vi "Allow UI_Write.vi"(8 "error in (no error)":errorcluster, 10 "Allow UI?":bool=TRUE, 11 "Dependency Source in":refnum<class "Dependency Source.lvclass">) -> (0 "error out":errorcluster, 3 "Dependency Source out":refnum<class "Dependency Source.lvclass">)   [LabVIEW 2019, in "Project.Dependencies Finder.lvlib" / "Dependency Source.lvclass"]
uses:
  Dependency Source.lvclass
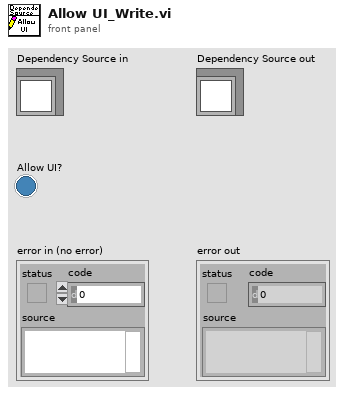
[diagram p1: front panel]
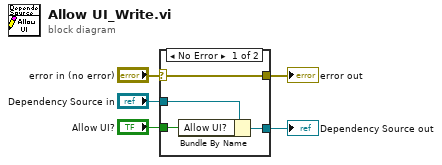
[diagram p0: block diagram]
diagram:
  n1 = case shown="No Error" "error in (no error)" {
    selector: "error in (no error)" -> [w9 w10]
    tunnel: [w9 w10] -> w4
    tunnel: [w7 w11] -> w2
    tunnel: "Dependency Source in" -> [w8 w11]
    tunnel: "Allow UI?" -> [w6 _]
    frame No Error {
      n2 = Bundle By Name(cluster=w8, "Allow UI?"=w6) -> (w7:refnum<class "Dependency Source.lvclass">)
    }
    frame Error {
    }
  }
  "error out" <- w4
  "Dependency Source out" <- w2
